vi "Read NChan 1Samp 1D SGL.vi"(8 "error in (no error)":errorcluster, 11 "MicroDAQ.lvlib:Analog Input.lvclass":refnum<class "Analog Input.lvclass">) -> (0 "error out":errorcluster, 2 "Values":dbl[](array[numeric]), 3 "MicroDAQ.lvlib:Analog Input.lvclass out":refnum<class "Analog Input.lvclass">)   [LabVIEW 2009, in "MicroDAQ.lvlib" / "Analog Input.lvclass"]
doc: "Reads a single floating-point sample from each channel."
uses:
  <instrlib>/MicroDAQ/Channel/Analog Input/Analog Input.lvclass
  <instrlib>/MicroDAQ/Channel/Analog Input/Analog Input.lvclass/Analog Input.ctl
  <instrlib>/MicroDAQ/Channel/Channel.lvclass
  <instrlib>/MicroDAQ/Mlink library wraper/mlink.lvlib
  <instrlib>/MicroDAQ/MicroDAQ.lvlib
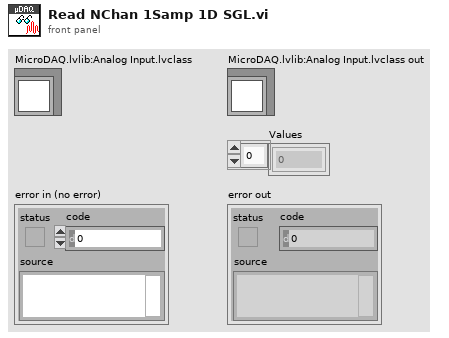
[diagram p1: front panel]
types:
  T1 = typedef "MicroDAQ.lvlib/Analog input type enum.ctl" = enum8{"Single-ended", "Differential"}
  T2 = typedef "MicroDAQ.lvlib/Analo Range Enum.ctl" = enum16{"±10V", "0-10V", "±5V", "0-5V", "±5.12V", "±2.56V", "±2.5V", "±2V", "±1.24V", "±0.64V"}
  T3 = typedef "MicroDAQ.lvlib/Analog input Channel enum.ctl" = u16
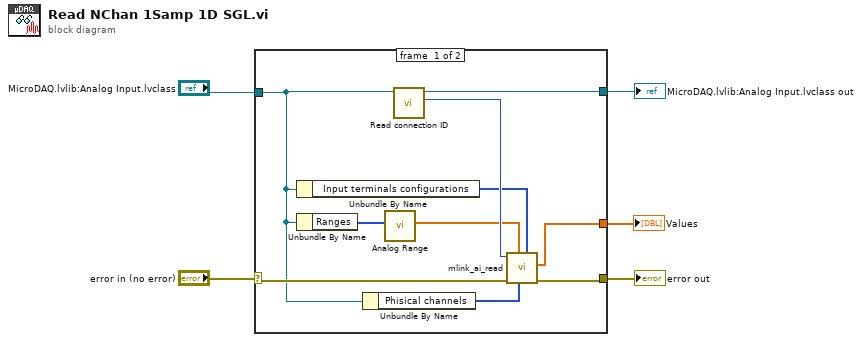
[diagram p0: block diagram]
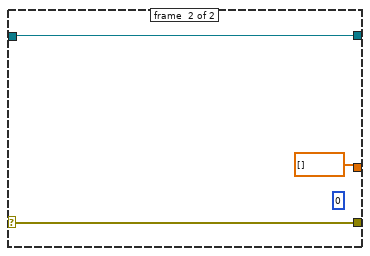
[diagram p2: hidden frame]
diagram:
  n1 = case shown="No Error" "error in (no error)" {
    selector: "error in (no error)" -> [w14 w17]
    tunnel: [w13 w17] -> w4
    tunnel: [w15 w18] -> w3
    tunnel: "MicroDAQ.lvlib:Analog Input.lvclass" -> [w8 w18]
    tunnel: [w6 dbl[] [] ("Values")] -> w1
    frame #0 {
      n2 = Unbundle By Name(w8) -> ("Input terminals configurations"=w7:T1[])
      n3 = Unbundle By Name(w8) -> ("Ranges"=w10:T2[])
      n4 = Unbundle By Name(w8) -> ("Phisical channels"=w11:T3[])
      n5 = call <instrlib>:"Analog Range.vi"("ranges in"=w10) -> ("range Array out"=w9:dbl[])  [unwired: 10 in]
      n6 = call <instrlib>:"Read connection ID.vi"("Task in"=w8) -> ("connection ID"=w12:i32, "Task out"=w15:refnum<class "Analog Input.lvclass">)  [unwired: 9 in]
      n7 = call <instrlib>:"mlink_ai_read.vi"("mode"=w7, "channels"=w11, "range"=w9, "error in (no error)"=w14, "connection ID"=w12) -> ("error out"=w13:errorcluster, "data out"=w6:dbl[])  [unwired: 4 in, 1 out]
    }
    frame #1 {
      (unwired) 0 ("read samples")
    }
  }
  "error out" <- w4
  "MicroDAQ.lvlib:Analog Input.lvclass out" <- w3
  "Values" <- w1
